vi "Save_Info.vi"(8 "error in (no error)":errorcluster, 11 "AB_Targetfile in":refnum<class "AB_Targetfile.lvclass">) -> (0 "error out":errorcluster, 3 "AB_Targetfile out":refnum<class "AB_Targetfile.lvclass">)   [LabVIEW 2020, in "AB_Targetfile.lvclass"]
uses:
  <vilib>/AppBuilder/AB_Classes/TargetFile/AB_Targetfile.lvclass
  e:/builds/penguin/labview/branches/2020/dev/dist/vi.lib/AppBuilder/AB_Classes/Build/AB_Build.lvclass
  <vilib>/AppBuilder/RW_Project/AB_RW_Project_PropBag_Action.ctl
  <vilib>/AppBuilder/RW_Project/AB_RW_Project_TargetFile_Data.ctl
  <vilib>/AppBuilder/AB_Classes/TargetFile/AB_Targetfile.lvclass/AB_Targetfile.ctl
  <vilib>/AppBuilder/AB_Classes/Build/AB_Build.lvclass
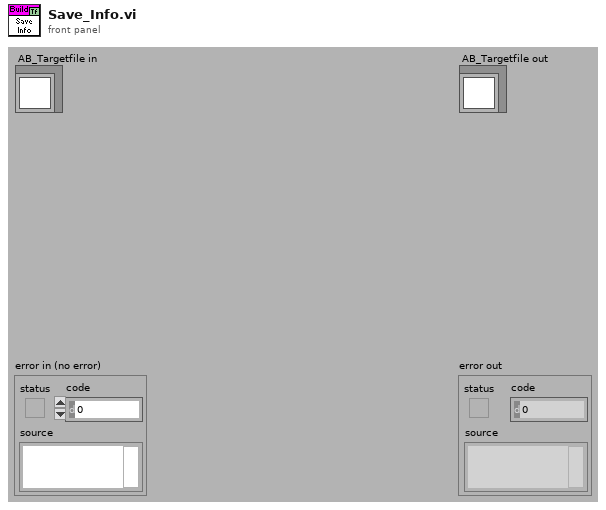
[diagram p1: front panel]
types:
  T1 = typedef "AB_RW_Project_PropBag_Action.ctl" = enum16{"read", "write", "clear", "readPrevious", "writePrevious", "clearPrevious"}
  T2 = typedef "AB_RW_Project_TargetFile_Data.ctl" = cluster{"targetfileName":string, "targetfileGUID":string, "enableDebugging":bool, "productName":string, "legalCopyright":string, "companyName":string, "internalName":string, "fileDescription":string, "eng_topLevelVI_DestinationPaths":path[], "fastFileFormat":bool, "versionIndependent":bool}
  T3 = typedef "AB_Build.ctl" = cluster{"buildSpecName":string, "buildSpecDescription":string, "destinations":refnum<class "AB_Destination.lvclass">[], "exclusionOption":T4, "defaultLanguage":string, "supportedLanguages":string[], "excludedDirectories":path[], "buildContext":refnum<vi>, "buildObject":T5, "preview":bool, "programatic":bool, "progressBarEvents":T6, "userLog_Path":path, "preActionID":string, "preAction_Path":path, "postActionID":string, "postAction_Path":path, "eng_checkForBrokenVIs?":bool, "eng_verboseLinkerErrors?":bool, "localDest_Path":path, "targetDest_Path":path, "removeVIObject":u16, "cache":refnum<class "PreviewCache.lvclass">, "use cache":bool, "previewCache_ID":string, "buildCache_ID":string, "eng_TempLocalDest_Path":path, "eng_collectDependencies?":bool, "versionInfo":cluster{"buildVersion":cluster{"major":u16, "minor":u16, "patch":u16, "build":u16}, "autoIncrement":bool}, "eng_enableVIChecksums":bool}
  T4 = typedef "AB_Exclusion_Option.ctl" = cluster{"typedefs":bool, "polymorphicVIs":bool, "unusedLibraryItems":bool, "modifyLibraryFile":bool, "edit-timeDependencies":bool, "inlineVIs":bool, "dependent PPLs":bool, "dependent DLLs":bool}
  T5 = typedef "ItemRef.ctl" = u64
  T6 = typedef "provcom_ProgressBar_Events.ctl" = cluster{"newJob":refnum<user-event>, "newItem":refnum<user-event>, "errorMsg":T7, "cancel":refnum<user-event>}
  T7 = typedef "mxLvBuildError.ctl" = refnum<user-event>
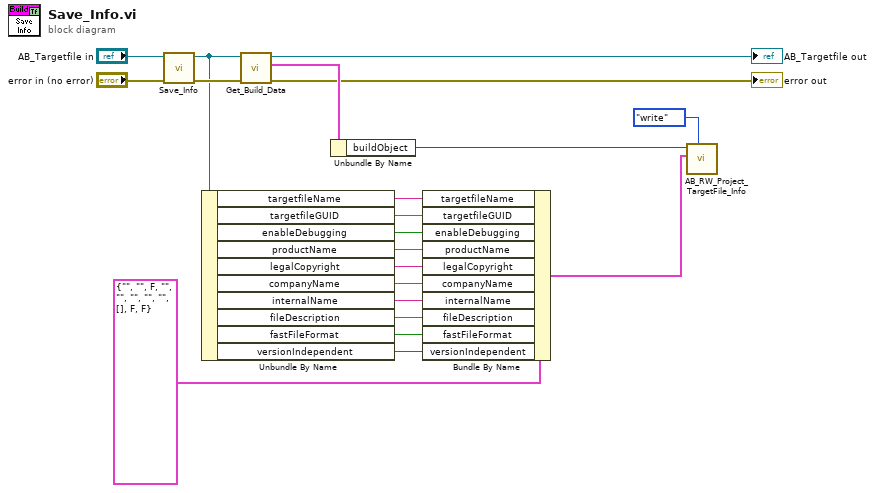
[diagram p0: block diagram]
diagram:
  n1 = call-parent "Save_Info.vi"("error in (no error)"="error in (no error)", "AB_Build in"="AB_Targetfile in") -> ("error out"=w17:errorcluster, "AB_Build out"=w15:refnum<class "AB_Targetfile.lvclass">)  [unwired: 8 in]
  n2 = Unbundle By Name(w15) -> ("targetfileName"=w13:string, "targetfileGUID"=w12:string, "enableDebugging"=w11:bool, "productName"=w10:string, "legalCopyright"=w9:string, "companyName"=w8:string, "internalName"=w7:string, "fileDescription"=w6:string, "fastFileFormat"=w2:bool, "versionIndependent"=w1:bool)
  n3 = call <vilib>:"Get_Build_Data.vi"("error in (no error)"=w17, "Class in"=w15) -> ("error out"=→"error out":errorcluster, "data"=w19:T3, "Class out"=→"AB_Targetfile out":refnum<class "AB_Targetfile.lvclass">)  [unwired: 7 out]
  n4 = Unbundle By Name(w19) -> ("buildObject"=w3:T5)
  n5 = Bundle By Name(cluster=T2 {"targetfileName"="", "targetfileGUID"="", "enableDebugging"=FALSE, "productName"="", "legalCopyright"="", "companyName"="", "internalName"="", "fileDescription"="", "eng_topLevelVI_DestinationPaths"=[], "fastFileFormat"=FALSE, "versionIndependent"=FALSE} ("targetfile info"), "targetfileName"=w13, "targetfileGUID"=w12, "enableDebugging"=w11, "productName"=w10, "legalCopyright"=w9, "companyName"=w8, "internalName"=w7, "fileDescription"=w6, "fastFileFormat"=w2, "versionIndependent"=w1) -> (w5:T2)
  n6 = call <vilib>:"AB_RW_Project_TargetFile_Info.vi"("action"=AB_RW_Project_PropBag_Action."write", "targetfileInfo in"=w5, "Object In"=w3) -> ()  [unwired: 6 in, 3 out]
